vi "Toroidal_rectifier_on.vi"   [LabVIEW 2015, in "Steps.lvlib"]
uses:
  Step_Vis/Steps.lvlib
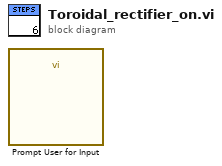
[diagram p0: block diagram]
diagram:
  n1 = call "Prompt User for Input"() -> ()  [unwired: 18 in, 2 out]
